vi "conc_state_args.vi"(0 "State":string, 7 "DELIMITER (:)":string=":", 11 "Args":string) -> (8 "state_and_args":string)   [LabVIEW 2021]
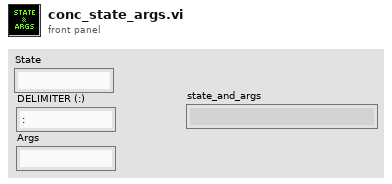
[diagram p1: front panel]
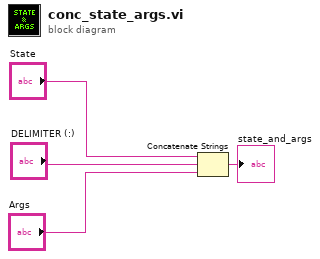
[diagram p0: block diagram]
diagram:
  n1 = Concatenate Strings("State", "DELIMITER (:)", "Args") -> (→"state_and_args":string)
